vi "Sections.vi"(8 "error in (no error)":errorcluster, 11 "Ini Path in":path) -> (0 "error out":errorcluster, 2 "All Sections":T1(array[cluster]), 3 "Ini Path out":path)   [LabVIEW 2018, in "Cfg.lvlib"]
uses:
  Cfg.lvlib
  Operation.ctl
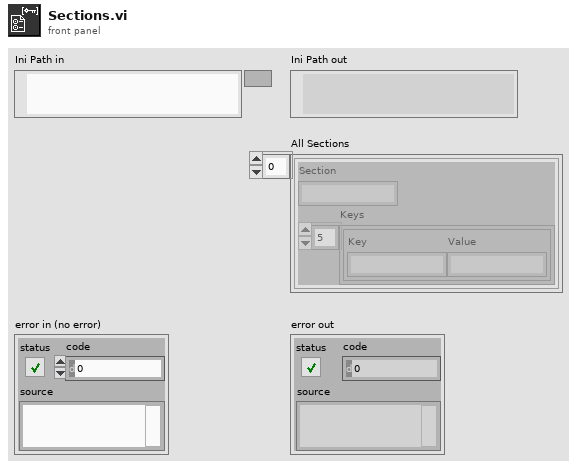
[diagram p1: front panel]
types:
  T1 = cluster{"Section":string, "Keys":cluster{"Key":string, "Value":string}[]}[]
  T2 = cluster{"Section":string, "Keys":cluster{"Key":string, "Value":string}[]}
  T3 = typedef "Cfg.lvlib/Operation.ctl" = enum8{"Read or Create", "Read", "Write"}
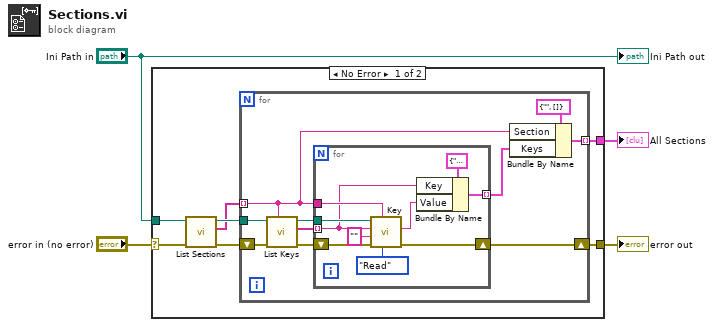
[diagram p0: block diagram]
diagram:
  n1 = case shown="No Error" "error in (no error)" {
    selector: "error in (no error)" -> [w11 w32]
    tunnel: "Ini Path in" -> [w10 _]
    tunnel: [w7 w32] -> w2
    tunnel: [w5 _] -> w1
    frame No Error {
      n2 = call "List Sections.vi"("error in (no error)"=w11, "Ini Path in"=w10) -> ("error out"=w9:errorcluster, "Sections"=w6:string[], "Ini Path out"=w8:path)  [unwired: 7 in]
      n3 = for {
        tunnel: w8 -> [w20]
        tunnel: w6 -> [w15] mode=indexing
        shift-right: [w18] -> w7
        shift-left: w9 -> [w21]
        tunnel: [w12] -> w5 mode=indexing
        n4 = call "List Keys.vi"("Section"=w15, "error in (no error)"=w21, "Ini Path in"=w20) -> ("error out"=w19:errorcluster, "Keys"=w16:string[], "Ini Path out"=w17:path)  [unwired: 5 in, 1 out]
        n5 = for {
          tunnel: w17 -> [w29]
          tunnel: w15 -> [w28]
          shift-right: [w30] -> w18
          shift-left: w19 -> [w31]
          tunnel: w16 -> [w24] mode=indexing
          tunnel: [w22] -> w13 mode=indexing
          n6 = call "Key.vi"("Operation (Read or Create)"=Operation."Read", "Section"=w28, "error in (no error)"=w31, "Value"="", "Key"=w24, "Ini Path in"=w29) -> ("error out"=w30:errorcluster, "Value out"=w23:string)  [unwired: 2 in, 2 out]
          n7 = Bundle By Name(cluster=cluster{"Key":string, "Value":string} {"Key"="", "Value"=""} ("Key"), "Key"=w24, "Value"=w23) -> (w22:cluster{"Key":string, "Value":string})
        }
        n8 = Bundle By Name(cluster=T2 {"Section"="", "Keys"=[]} ("Section"), "Section"=w15, "Keys"=w13) -> (w12:T2)
      }
    }
    frame Error {
    }
  }
  "error out" <- w2
  "All Sections" <- w1
  "Ini Path out" <- "Ini Path in"
